vi "add date n count in sequence.vi"(8 "find date":string[](array[string]), 9 "total date":string[](array[string]), 10 "duration":dbl[](array[numeric])=[222.0], 11 "count":dbl[](array[numeric])=[222.0]) -> (1 "DURATION":string[](array[string]), 2 "COUNT":string[](array[string]), 3 "appended array":string[][](array[string]))   [LabVIEW 2017]
panel:
  out "output array 2":dbl[](array[numeric])
  out "output array":dbl[](array[numeric])
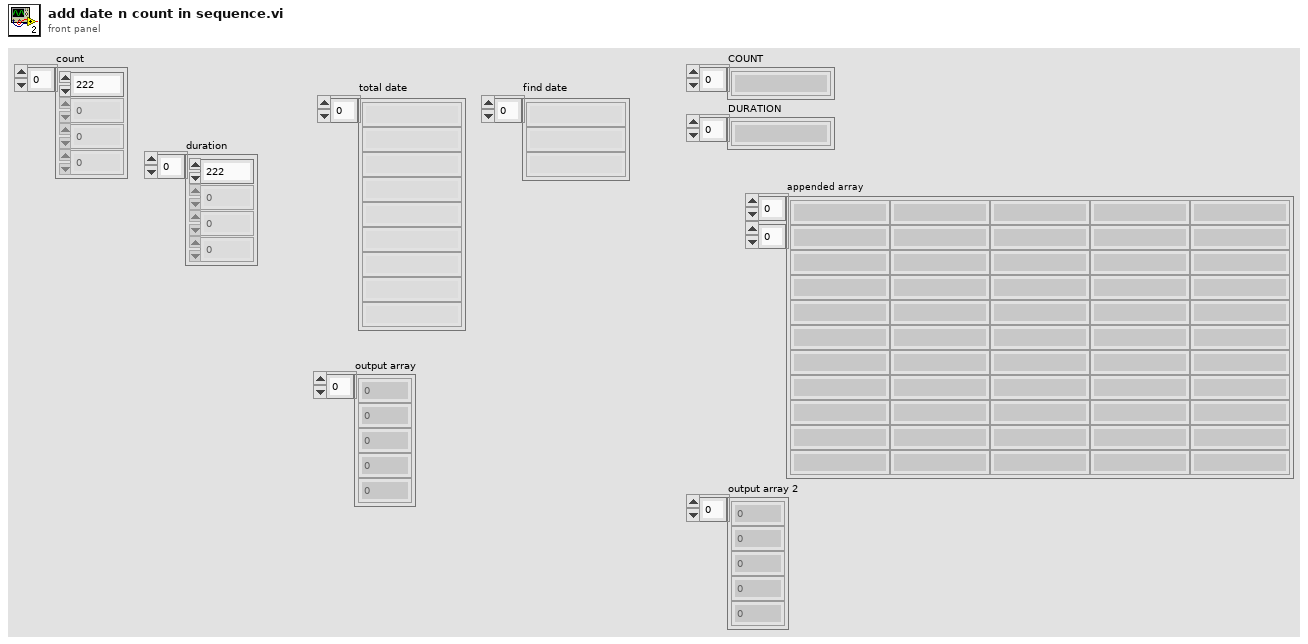
[diagram p1: front panel]
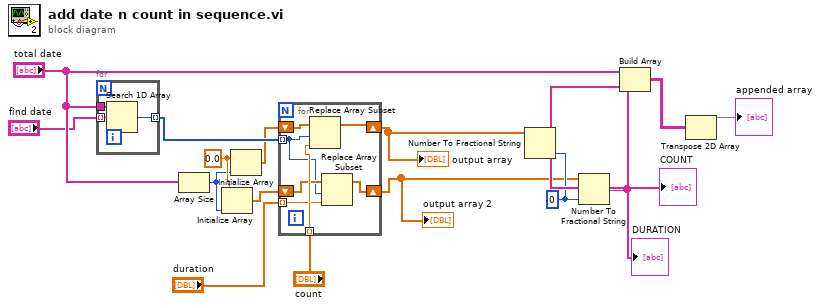
[diagram p0: block diagram]
diagram:
  w7 = i16 0 ("precision (6)")
  w4 = 0.0 ("element")
  n1 = for {
    tunnel: [w19] -> w16 mode=indexing
    tunnel: "total date" -> [w18]
    tunnel: "find date" -> [w17] mode=indexing
    n2 = Search 1D Array(1D array=w18, element=w17) -> (index of element=w19:i32)  [unwired: 1 in]
  }
  n3 = Array Size(array="total date") -> (size(s)=w3:i32)
  n4 = Initialize Array(w4, w3) -> (w5:dbl[])
  n5 = Initialize Array(w4, w3) -> (w11:dbl[])
  n6 = for {
    tunnel: w16 -> [w20] mode=indexing
    shift-right: [w25] -> w9
    shift-left: w11 -> [w26]
    tunnel: "count" -> [w24] mode=indexing
    shift-right: [w21] -> w1
    shift-left: w5 -> [w23]
    tunnel: "duration" -> [w22] mode=indexing
    n7 = Replace Array Subset(array=w26, new element=w24, index=w20) -> (w25:dbl[])
    n8 = Replace Array Subset(array=w23, new element=w22, index=w20) -> (w21:dbl[])
  }
  "output array" <- w9
  "output array 2" <- w1
  n9 = Number To Fractional String(number=w9, precision (6)=w7) -> (F-format string=w15:string[])  [unwired: 2 in]
  "COUNT" <- w15
  n10 = Number To Fractional String(number=w1, precision (6)=w7) -> (F-format string=w6:string[])  [unwired: 2 in]
  "DURATION" <- w6
  n11 = Build Array("total date", w15, w6) -> (w13:string[][])
  n12 = Transpose 2D Array(2D array=w13) -> (transposed array=→"appended array":string[][])
